vi "LEP_RV_LaunchRun.vi"(8 "error in (no error)":errorcluster, 9 "action":T1) -> (0 "error out":errorcluster)   [LabVIEW 2011]
doc: "Runs the embedded application on a console located in the <B>Build Path</B> directory ."
uses:
  <vilib>/Platform/EmbProject/utilities/Emb_Utility_AppAction.ctl
  <vilib>/LabVIEW Targets/Embedded/ASWServer/MPU_ASWServer_Messages.ctl
  <vilib>/LabVIEW Targets/Embedded/ASWServer/MPU_ASWServer_GeneralIcons.ctl
  <vilib>/LabVIEW Targets/Embedded/ASWServer/MPU_ASWServer_GeneralCtrls.ctl
  LEP_RV_LaunchGlobals.vi
  <vilib>/LabVIEW Targets/Embedded/ASWServer/MPU_ASWServer_General_SetProgressBarTitle.vi
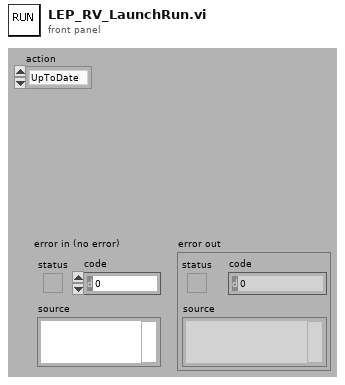
[diagram p1: front panel]
types:
  T1 = typedef "Emb_Utility_AppAction.ctl" = enum16{"UpToDate", "Build", "Cancel", "Error"}
  T2 = typedef "MPU_ASWServer_Messages.ctl" = enum32{"NoMessage", "Cancel", "ApplicationLaunched"}
  T3 = typedef "LEP_RV_Config.ctl" = cluster{"Enable debugging":bool, "Debug Options":u16, "Use stack variables":bool, "Generate serial only":bool, "Generate guard code":bool, "Generate Integer Only":bool, "Generate C Function Calls":bool, "ExpressionFolding":bool, "Constant Allocation":u16, "Constant Deallocation":u16, "Build Specification ID":string, "Preprocessor symbols (define)":string, "Compiler Flags":string, "Linker Flags":string, "Mode":u16, "Optimization":u16, "Optimize for time":bool, "Enable cross-module optimization":bool, "Include paths":path[], "Optimize heap size":bool, "Use MicroLib":bool, "Debug Mode":u16, "Enable profile information":bool, "Host name":string, "Use DHCP":bool, "IP address":string, "Subnet mask":string, "Gateway":string, "Primary DNS":string, "Secondary DNS":string, "MAC in target memory":bool, "MAC address":string, "Console output":u16, "Target serial port":u16}
  T4 = typedef "MPU_ASWServer_GeneralIcons.ctl" = enum16{"Complete", "Disconnected", "Error", "Initializing", "Ready", "Running", "Stopped", "Unknown", "No Change"}
  T5 = typedef "MPU_ASWServer_GeneralCtrls.ctl" = enum16{"Build Status", "Download Status", "Target Name", "Target Type", "Application Name"}
  T6 = enum16{"Normal", "Minimized", "Maximized", "Hidden", "Locked"}
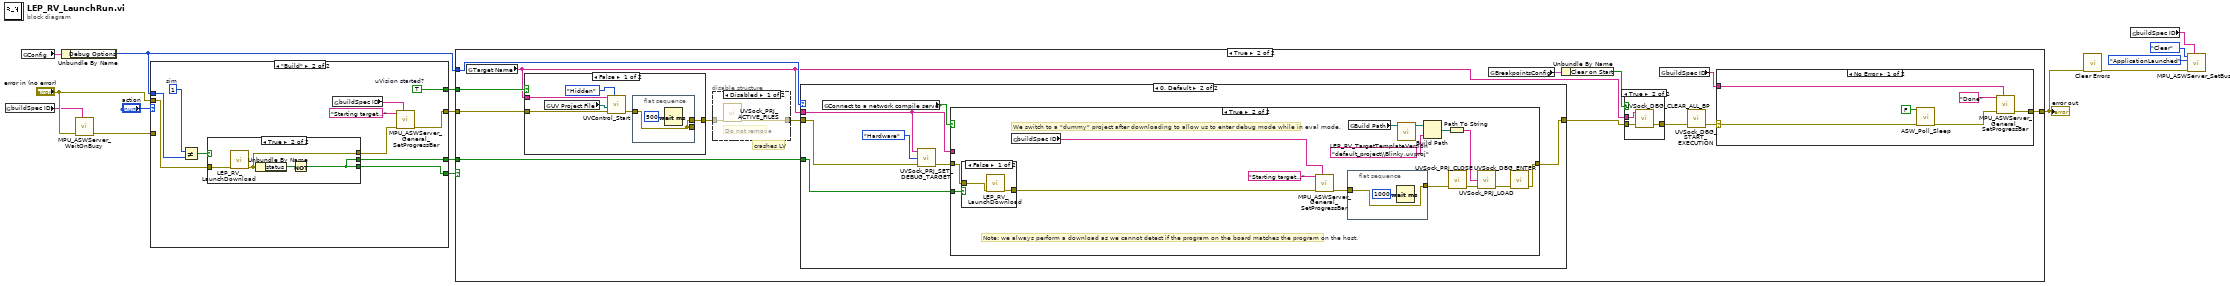
[diagram p0: block diagram]
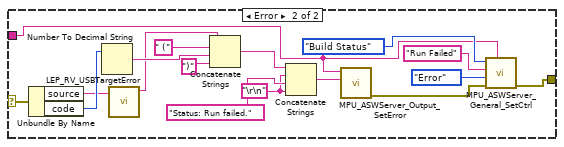
[diagram p4: hidden frame]
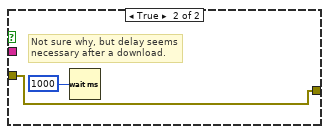
[diagram p6: hidden frame]
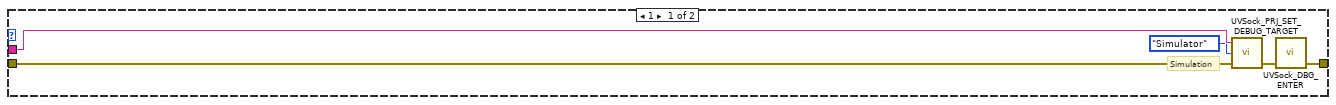
[diagram p7: hidden frame]
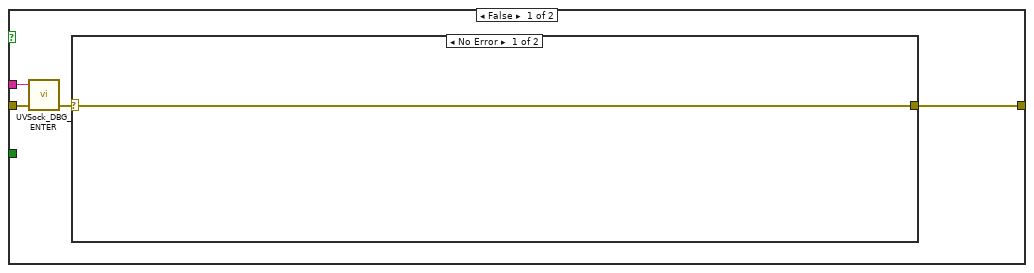
[diagram p8: hidden frame]
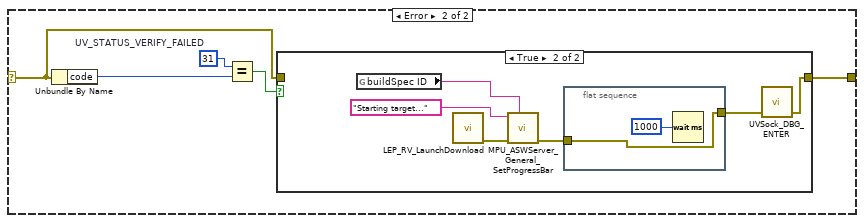
[diagram p9: hidden frame]
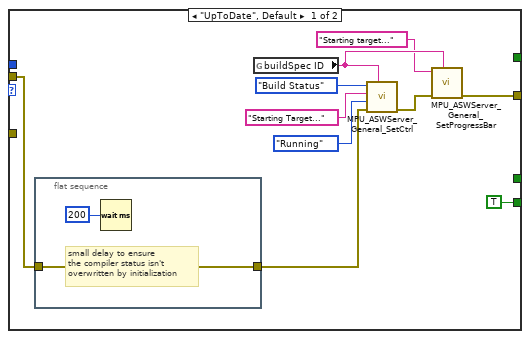
[diagram p12: hidden frame]
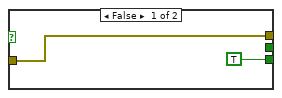
[diagram p13: hidden frame]
diagram:
  n1 = global read "LEP_RV_LaunchGlobals.vi" "buildSpec ID"() -> (w8:string)
  n2 = global read "LEP_RV_LaunchGlobals.vi" "Config"() -> (w10:T3)
  n3 = Unbundle By Name(w10) -> ("Debug Options"=w13:u16)
  n4 = call <vilib>:"MPU_ASWServer_WaitOnBusy.vi"("buildSpec ID"=w8, "error in"="error in (no error)") -> ("error out"=w7:errorcluster)  [unwired: 9 out]
  n5 = case shown="\"Build\"" "action" {
    tunnel: [TRUE w38] -> w14
    tunnel: "error in (no error)" -> [w17 w34]
    tunnel: [w18 w30] -> w15
    tunnel: [_ w37] -> w12
    tunnel: w13 -> [_ w36]
    tunnel: w7 -> [_ _]
    tunnel: [_ w28] -> w1
    frame "UpToDate", Default {
      n6 = flat-sequence {
        tunnel: w17 -> [w27]
        tunnel: [w27] -> w16
        frame #0 {
          # "small delay to ensure\nthe compiler status isn't \noverwritten by initialization"
          n7 = Wait (ms)(milliseconds to wait=u32 200) -> ()  [unwired: 1 out]
        }
      }
      n8 = global read "LEP_RV_LaunchGlobals.vi" "buildSpec ID"() -> (w20:string)
      n9 = call <vilib>:"MPU_ASWServer_General_SetCtrl.vi"("buildSpec ID"=w20, "error in"=w16, "icon"=MPU_ASWServer_GeneralIcons."Running", "value"="Starting Target...", "control"=MPU_ASWServer_GeneralCtrls."Build Status") -> ("error out"=w21:errorcluster)  [unwired: 4 in, 2 out]
      n10 = call-poly <vilib>:"MPU_ASWServer_General_SetProgressBar.vi"("buildSpec ID"=w20, "error in"=w21, "title"="Starting target...") -> ("error out"=w18:errorcluster)  [unwired: 6 in, 2 out]
    }
    frame "Build" {
      w35 = u16 1  # sim
      w37 = TRUE  # uVision started?
      n11 = Not Equal?(x=w35, y=w36) -> (x != y?=w33:bool)
      n12 = case shown="True" w33 {
        tunnel: [w40 w42] -> w31
        tunnel: [TRUE w41] -> w38
        tunnel: w34 -> [w40 w43]
        tunnel: [_ w41] -> w28
        frame False {
        }
        frame True {
          n13 = call "LEP_RV_LaunchDownload.vi"("error in (no error)"=w43) -> ("error out"=w42:errorcluster)  [unwired: 10 in]
          n14 = Unbundle By Name(w42) -> ("status"=w44:bool)
          n15 = Not(x=w44) -> (.not. x?=w41:bool)
        }
      }
      n16 = global read "LEP_RV_LaunchGlobals.vi" "buildSpec ID"() -> (w29:string)
      n17 = call-poly <vilib>:"MPU_ASWServer_General_SetProgressBar.vi"("buildSpec ID"=w29, "error in"=w31, "title"="Starting target...") -> ("error out"=w30:errorcluster)  [unwired: 6 in, 2 out]
    }
  }
  n18 = case shown="True" w14 {
    tunnel: w15 -> [w45 w56]
    tunnel: [w45 w54] -> w6
    tunnel: w12 -> [_ w53]
    tunnel: w13 -> [_ w57]
    tunnel: w1 -> [_ w46]
    frame False {
    }
    frame True {
      # "crashes LV"
      n19 = global read "LEP_RV_LaunchGlobals.vi" "Target Name"() -> (w52:string)
      n20 = case shown="False" w53 {
        tunnel: w56 -> [w92 w99]
        tunnel: w52 -> [w95 _]
        tunnel: [w91 w99] -> w49
        frame False {
          n21 = global read "LEP_RV_LaunchGlobals.vi" "UV Project File"() -> (w90:path)
          n22 = call "UVControl_Start.vi"("Mode"=T6."Hidden", "error in (no error)"=w92, "Project File"=w90, "Target"=w95) -> ("error out"=w93:errorcluster)  [unwired: 1 in, 6 out]
          n23 = flat-sequence {
            tunnel: w93 -> [w96]
            tunnel: [w96] -> _
            tunnel: [w96] -> w91
            frame #0 {
              n24 = Wait (ms)(milliseconds to wait=u32 500) -> ()  [unwired: 1 out]
            }
          }
        }
        frame True {
          # "Not sure why, but delay seems necessary after a download."
          n25 = Wait (ms)(milliseconds to wait=u32 1000) -> ()  [unwired: 1 out]
        }
      }
      n26 = disable-structure shown="Disabled" {
        disable-tunnel: [w61 w62] -> w55
        disable-tunnel: w49 -> [w60 w62]
        frame Disabled {
          # "Do not remove"
          n27 = call "UVSock_PRJ_ACTIVE_FILES.vi"("error in (no error)"=w60) -> ("error out"=w61:errorcluster)  [unwired: 1 in, 5 out]
        }
        frame Enabled {
        }
      }
      n28 = case shown="0, Default" w57 {
        tunnel: w55 -> [w102 w107]
        tunnel: [w103 w108] -> w59
        tunnel: w52 -> [w101 w110]
        tunnel: w46 -> [_ w106]
        frame 1 {
          # "Simulation"
          n29 = call "UVSock_PRJ_SET_DEBUG_TARGET.vi"("error in (no error)"=w102, "Debug Target"=enum16{"Hardware", "Simulator"}."Simulator", "Target"=w101) -> ("error out"=w104:errorcluster)  [unwired: 2 out]
          n30 = call "UVSock_DBG_ENTER.vi"("error in (no error)"=w104) -> ("error out"=w103:errorcluster)  [unwired: 1 in, 3 out]
        }
        frame 0, Default {
          n31 = global read "LEP_RV_LaunchGlobals.vi" "Connect to a network compile server"() -> (w105:bool)
          n32 = call "UVSock_PRJ_SET_DEBUG_TARGET.vi"("error in (no error)"=w107, "Debug Target"=enum16{"Hardware", "Simulator"}."Hardware", "Target"=w110) -> ("error out"=w111:errorcluster)  [unwired: 2 out]
          n33 = case shown="True" w105 {
            tunnel: w111 -> [w114 w141]
            tunnel: w110 -> [w113 _]
            tunnel: [w112 w140] -> w108
            tunnel: w106 -> [_ w132]
            frame False {
              n34 = call "UVSock_DBG_ENTER.vi"("error in (no error)"=w114, "Target"=w113) -> ("error out"=w115:errorcluster)  [unwired: 3 out]
              n35 = case shown="No Error" w115 {
                selector: w115 -> [w116 w118]
                tunnel: [w116 w117] -> w112
                frame No Error {
                }
                frame Error {
                  w120 = 31  # UV_STATUS_VERIFY_FAILED
                  n36 = Unbundle By Name(w118) -> ("code"=w121:i32)
                  n37 = Equal?(x=w120, y=w121) -> (x = y?=w119:bool)
                  n38 = case shown="True" w119 {
                    tunnel: w118 -> [w122 _]
                    tunnel: [w122 w127] -> w117
                    frame False {
                    }
                    frame True {
                      n39 = global read "LEP_RV_LaunchGlobals.vi" "buildSpec ID"() -> (w126:string)
                      n40 = call "LEP_RV_LaunchDownload.vi"() -> ("error out"=w124:errorcluster)  [unwired: 11 in]
                      n41 = call-poly <vilib>:"MPU_ASWServer_General_SetProgressBar.vi"("buildSpec ID"=w126, "error in"=w124, "title"="Starting target...") -> ("error out"=w123:errorcluster)  [unwired: 6 in, 2 out]
                      n42 = flat-sequence {
                        tunnel: w123 -> [w129]
                        tunnel: [w129] -> w128
                        frame #0 {
                          n43 = Wait (ms)(milliseconds to wait=u32 1000) -> ()  [unwired: 1 out]
                        }
                      }
                      n44 = call "UVSock_DBG_ENTER.vi"("error in (no error)"=w128) -> ("error out"=w127:errorcluster)  [unwired: 1 in, 3 out]
                    }
                  }
                }
              }
            }
            frame True {
              # "Note: we always perform a download as we cannot detect if the program on the board matches the program on the host."
              # "We switch to a \"dummy\" project after downloading to allow us to enter debug mode while in eval mode."
              n45 = case shown="False" w132 {
                tunnel: [w147 w148] -> w143
                tunnel: w141 -> [w146 w148]
                frame False {
                  n46 = call "LEP_RV_LaunchDownload.vi"("error in (no error)"=w146) -> ("error out"=w147:errorcluster)  [unwired: 10 in]
                }
                frame True {
                }
              }
              n47 = global read "LEP_RV_LaunchGlobals.vi" "buildSpec ID"() -> (w145:string)
              n48 = call-poly <vilib>:"MPU_ASWServer_General_SetProgressBar.vi"("buildSpec ID"=w145, "error in"=w143, "title"="Starting target...") -> ("error out"=w142:errorcluster)  [unwired: 6 in, 2 out]
              n49 = flat-sequence {
                tunnel: w142 -> [w149]
                tunnel: [w149] -> w138
                frame #0 {
                  n50 = Wait (ms)(milliseconds to wait=u32 1000) -> ()  [unwired: 1 out]
                }
              }
              n51 = global read "LEP_RV_LaunchGlobals.vi" "Build Path"() -> (w134:path)
              n52 = call "LEP_RV_TargetTemplateVersion.vi"("Path"=w134) -> ("Path plus Version"=w133:path)  [unwired: 8 in, 2 out]
              n53 = Build Path(base path=w133, name or relative path="default_project\\Blinky.uvproj") -> (appended path=w137:path)
              n54 = Path To String(path=w137) -> (string=w135:string)
              n55 = call "UVSock_PRJ_CLOSE.vi"("error in (no error)"=w138) -> ("error out"=w131:errorcluster)  [unwired: 4 in]
              n56 = call "UVSock_PRJ_LOAD.vi"("error in (no error)"=w131, "Project File"=w135) -> ("error out"=w139:errorcluster)  [unwired: 3 in]
              n57 = call "UVSock_DBG_ENTER.vi"("error in (no error)"=w139) -> ("error out"=w140:errorcluster)  [unwired: 1 in, 3 out]
            }
          }
        }
      }
      n58 = global read "LEP_RV_LaunchGlobals.vi" "BreakpointsConfig"() -> (w51:cluster{"Clear on Start":bool})
      n59 = Unbundle By Name(w51) -> ("Clear on Start"=w50:bool)
      n60 = case shown="True" w50 {
        tunnel: w52 -> [_ w89]
        tunnel: w59 -> [w86 w88]
        tunnel: [w86 w87] -> w58
        frame False {
        }
        frame True {
          n61 = call "UVSock_DBG_CLEAR_ALL_BP.vi"("error in (no error)"=w88, "Target"=w89) -> ("error out"=w87:errorcluster)  [unwired: 3 out]
        }
      }
      n62 = global read "LEP_RV_LaunchGlobals.vi" "buildSpec ID"() -> (w48:string)
      n63 = call "UVSock_DBG_START_EXECUTION.vi"("error in (no error)"=w58) -> ("error out"=w47:errorcluster)  [unwired: 1 in, 3 out]
      n64 = case shown="No Error" w47 {
        selector: w47 -> [w65 w74]
        tunnel: [w68 w75] -> w54
        tunnel: w48 -> [w66 w77]
        frame No Error {
          n65 = call <vilib>:"ASW_Poll_Sleep.vi"("Sleep"=FALSE ("Sleep?"), "error in (no error)"=w65) -> ("error out"=w64:errorcluster)  [unwired: 13 in]
          n66 = call-poly <vilib>:"MPU_ASWServer_General_SetProgressBar.vi"("buildSpec ID"=w66, "error in"=w64, "title"="Done") -> ("error out"=w68:errorcluster)  [unwired: 6 in, 2 out]
        }
        frame Error {
          w71 = "\r\n"
          n67 = Unbundle By Name(w74) -> ("source"=w70:string, "code"=w85:i32)
          n68 = Number To Decimal String(number=w85) -> (decimal integer string=w82:string)  [unwired: 1 out]
          n69 = call "LEP_RV_USBTargetError.vi"("source"=w70) -> ("source out"=w69:string)  [unwired: 10 in]
          n70 = Concatenate Strings(w69, " (" ("string"), w82, ")" ("string")) -> (w73:string)
          n71 = Concatenate Strings(w73, w71, "Status: Run failed." ("title"), w71) -> (w81:string)
          n72 = call <vilib>:"MPU_ASWServer_Output_SetError.vi"("error str"=w81, "buildSpec ID"=w77) -> ("error out"=w76:errorcluster)  [unwired: 7 in]
          n73 = call <vilib>:"MPU_ASWServer_General_SetCtrl.vi"("buildSpec ID"=w77, "error in"=w76, "icon"=MPU_ASWServer_GeneralIcons."Error", "value"="Run Failed", "control"=MPU_ASWServer_GeneralCtrls."Build Status") -> ("error out"=w75:errorcluster)  [unwired: 4 in, 2 out]
        }
      }
    }
  }
  "error out" <- w6
  n74 = call <vilib>:"Clear Errors.vi"("error in (no error)"=w6) -> ("error out"=w5:errorcluster)  [unwired: 6 in]
  n75 = global read "LEP_RV_LaunchGlobals.vi" "buildSpec ID"() -> (w4:string)
  n76 = call <vilib>:"MPU_ASWServer_SetBusy.vi"("buildSpec ID"=w4, "error in (no error)"=w5, "message"=MPU_ASWServer_Messages."ApplicationLaunched", "action"=enum32{"Clear", "Set"}."Clear") -> ()  [unwired: 6 out]
